vi "Servo MSMT ET Set Measurement Standard.vi"(8 "error in (no error)":errorcluster, 10 "Step In":refnum<k7>, 11 "Servo MSMT in":refnum<class "Servo MSMT.lvclass">) -> (0 "error out":errorcluster, 2 "Step Out":refnum<k7>, 3 "Servo MSMT out":refnum<class "Servo MSMT.lvclass">)   [LabVIEW 2018, in "Servo MSMT.lvlib" / "Servo MSMT.lvclass"]
uses:
  Servo MSMT.lvclass
  C:/Sequence Automation/Plugins/Measurement Interface.lvlibp/Measurement Interface.lvclass
  Plugins/Measurement Interface.lvlibp/Private Methods/Measurement Parameters/Read Measurement Parameters.vi
  Plugins/String Database.lvlibp/String Database.lvclass
  Plugins/TestStand API Tools (TSAT).lvlibp/Step Actions/TSAT Step Actions.lvlib
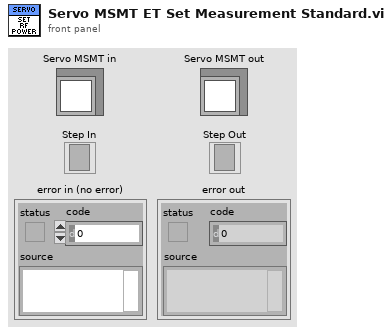
[diagram p1: front panel]
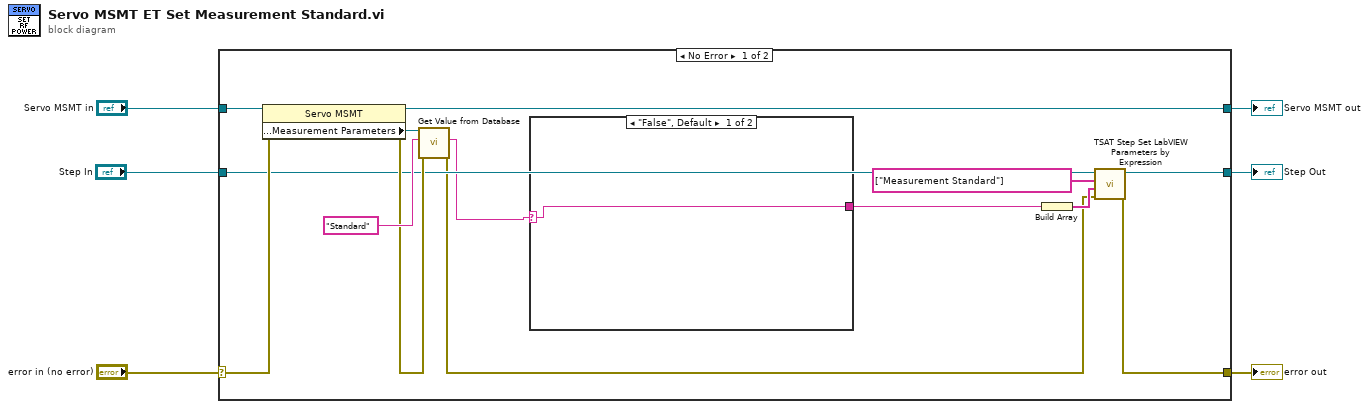
[diagram p0: block diagram]
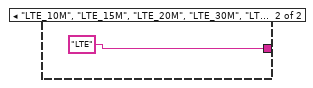
[diagram p2: hidden frame]
diagram:
  n1 = case shown="No Error" "error in (no error)" {
    selector: "error in (no error)" -> [w20 w25]
    tunnel: [w12 w25] -> w5
    tunnel: [w18 w24] -> w3
    tunnel: "Servo MSMT in" -> [w19 w24]
    tunnel: "Step In" -> [w14 w23]
    tunnel: [w13 w23] -> w1
    frame No Error {
      n2 = property class="Servo MSMT"(reference=w19, error in=w20) -> (reference out=w18:refnum<class "Servo MSMT.lvclass">, error out=w15:errorcluster, "Protected Methods:Measurement Parameters"=w17:refnum<class "String Database.lvclass">)
      n3 = call "Get Value from Database.vi"("error in (no error)"=w15, "Entry Name"="Standard", "Message in"=w17) -> ("error out"=w9:errorcluster, "Entry Value"=w8:string)  [unwired: 5 in, 2 out]
      n4 = case shown="\"False\", Default" w8 {
        selector: w8 -> [w21 _]
        tunnel: [w21 "LTE"] -> w7
        frame "False", Default {
        }
        frame "LTE_10M", "LTE_15M", "LTE_20M", "LTE_30M", "LTE_40M" {
        }
      }
      n5 = Build Array(w7) -> (w10:string[])
      n6 = call "TSAT Step Set LabVIEW Parameters by Expression.vi"("Error In"=w9, "Value Expressions"=w10, "Parameters to Set"=string[] ["Measurement Standard"], "Step In"=w14) -> ("Error Out"=w12:errorcluster, "Step Out"=w13:refnum<k7>)  [unwired: 6 in]
    }
    frame Error {
    }
  }
  "error out" <- w5
  "Servo MSMT out" <- w3
  "Step Out" <- w1
